vi "Get UUT Info.vi"(8 "error in (no error)":errorcluster, 10 "Scanned Only (false)":bool, 11 "Application in":refnum<class "Application.lvclass">) -> (0 "error out":errorcluster, 2 "All UUTs":T1(array[cluster]), 3 "Application out":refnum<class "Application.lvclass">)   [LabVIEW 2017, in "Application.lvlib" / "Application.lvclass"]
uses:
  Application.lvclass
  Application.lvclass/Application.ctl
  Properties/App Properties.lvclass
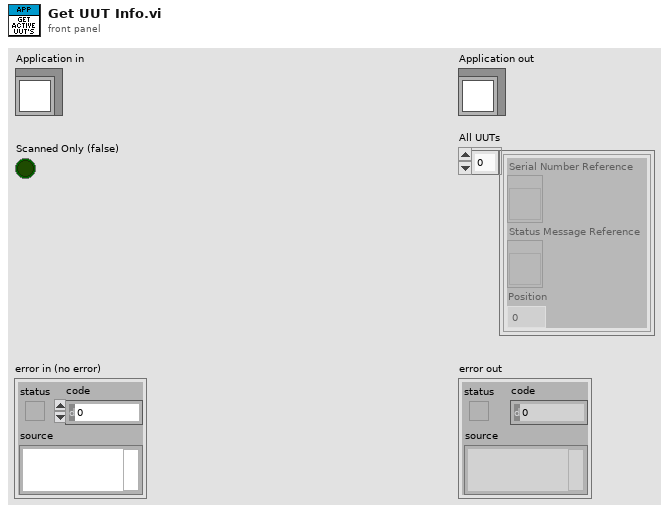
[diagram p1: front panel]
types:
  T1 = cluster{"Serial Number Reference":refnum<vi>, "Status Message Reference":refnum<vi>, "Position":u32}[]
  T2 = cluster{"Serial Number Reference":refnum<vi>, "Status Message Reference":refnum<vi>, "Position":u32}
  T3 = typedef "Application.lvlib/App Properties.lvclass/Class Properties -- Cluster.ctl" = cluster{"UUT Info":T4[], "Test Information":refnum<vi>, "Gold Board":refnum<class "Golden Board.lvclass">, "Test Recipe":refnum<class "Test Recipe.lvclass">, "Instruments":refnum<class "Instrument.lvclass">[], "Mode":T5, "Test Results":T6[], "Station Config":refnum<class "Station Config.lvclass">, "Variable Engine":refnum<class "Variable Engine.lvclass">}
  T4 = typedef "Application.lvlib/App Properties.lvclass/UUT Reference -- Cluster.ctl" = cluster{"Serial Number Reference":refnum<vi>, "Status Message Reference":refnum<vi>}
  T5 = typedef "Application.lvlib/Application.lvclass/Op Mode -- Enum.ctl" = u16
  T6 = typedef "Application.lvlib/App Properties.lvclass/Test Result -- Cluster.ctl" = cluster{"Position":i32, "Pass":bool, "Fail Codes":string}
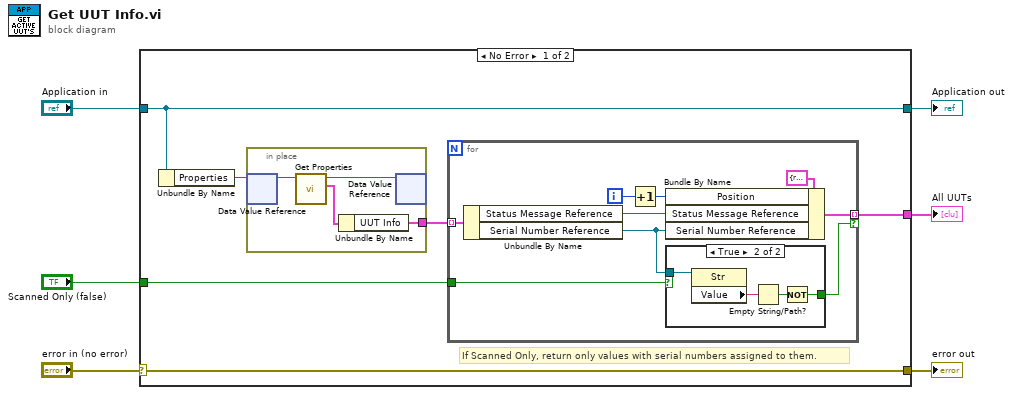
[diagram p0: block diagram]
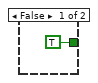
[diagram p2: hidden frame]
diagram:
  n1 = case shown="No Error" "error in (no error)" {
    selector: "error in (no error)" -> [w12 w32]
    tunnel: [w12 w32] -> w5
    tunnel: [w11 w31] -> w3
    tunnel: "Application in" -> [w11 w31]
    tunnel: [w8 _] -> w2
    tunnel: "Scanned Only (false)" -> [w7 _]
    frame No Error {
      # "If Scanned Only, return only values with serial numbers assigned to them."
      n2 = Unbundle By Name(w11) -> ("Properties"=w10:refnum<data-value>)
      n3 = in-place {
        in-place-border: [w27] -> w9
        n4 = in-place-dvr #1(w10) -> (w30:refnum<class "App Properties.lvclass">)  [unwired: 1 out]
        n5 = call-dynamic "Get Properties.vi"("App Properties in"=w30) -> ("Class Properties"=w28:T3, "App Properties out"=w29:refnum<class "App Properties.lvclass">)  [unwired: 8 in, 1 out]
        n6 = Unbundle By Name(w28) -> ("UUT Info"=w27:T4[])
        n7 = in-place-dvr #1(w29) -> ()  [unwired: 2 out]
      }
      n8 = for {
        tunnel: w9 -> [w21] mode=indexing
        tunnel: [w15] -> w8 mode=indexing if=w14
        tunnel: w7 -> [w13]
        i -> [w17]
        n9 = Unbundle By Name(w21) -> ("Status Message Reference"=w19:refnum<vi>, "Serial Number Reference"=w18:refnum<vi>)
        n10 = Increment(x=w17) -> (x+1=w16:i32)
        n11 = Bundle By Name(cluster=T2 {"Serial Number Reference"=refnum, "Status Message Reference"=refnum, "Position"=0} ("Active UUTs"), "Position"=w16, "Status Message Reference"=w19, "Serial Number Reference"=w18) -> (w15:T2)
        n12 = case shown="True" w13 {
          tunnel: w18 -> [_ w26]
          tunnel: [TRUE w23] -> w14
          frame False {
          }
          frame True {
            n13 = property class="Str"(reference=w26) -> ("Value"=w25:string)  [unwired: 1 in, 2 out]
            n14 = Empty String/Path?(string/path=w25) -> (empty?=w24:bool)
            n15 = Not(x=w24) -> (.not. x?=w23:bool)
          }
        }
      }
    }
    frame Error {
    }
  }
  "error out" <- w5
  "Application out" <- w3
  "All UUTs" <- w2
